vi "ggg.vi"() -> ()   [LabVIEW 2015]
uses:
  <vilib>/NXT/Block Support/NXT_InputPort.ctl
  <vilib>/NXT/Block Support/NXT_OutputPort.ctl
  <vilib>/NXT/Dual Mode Library/Sensors/Sonar_cm.vi
  <vilib>/NXT/Dual Mode Library/Sensors/Light_On.vi
  <vilib>/NXT/NXTIO Xnodes/NXTIONodeSubVIs/NXTMoveMotors.vi
  <vilib>/NXT/Dual Mode Library/Waits/Wait_Num.vi
  <vilib>/NXT/NXTIO Xnodes/AddressXNode/NXTIOAddress.xnode
  <vilib>/NXT/Subs/LVHSConnector.ctl
  <vilib>/NXT/NXTIO Xnodes/NXTIOXNode/NXTIO.xnode
  <vilib>/NXT/LegoClasses/BrickReference/BrickReference.lvclass
panel:
  in  "Port (Port 3) 4":T1=2 items=["Port 1", "Port 2", "Port 3", "Port 4"]
  in  "Port (Port 3) 3":T1=2 items=["Port 1", "Port 2", "Port 3", "Port 4"]
  in  "Power/Speed 1":i8=75
  in  "Port (Port 3) 2":T1=2 items=["Port 1", "Port 2", "Port 3", "Port 4"]
  in  "Port (Port 3)":T1=2 items=["Port 1", "Port 2", "Port 3", "Port 4"]
  in  "Power/Speed 3":i8=75
  in  "Port (Port 4)":T1=3 items=["Port 1", "Port 2", "Port 3", "Port 4"]
  in  "沥瘤":bool
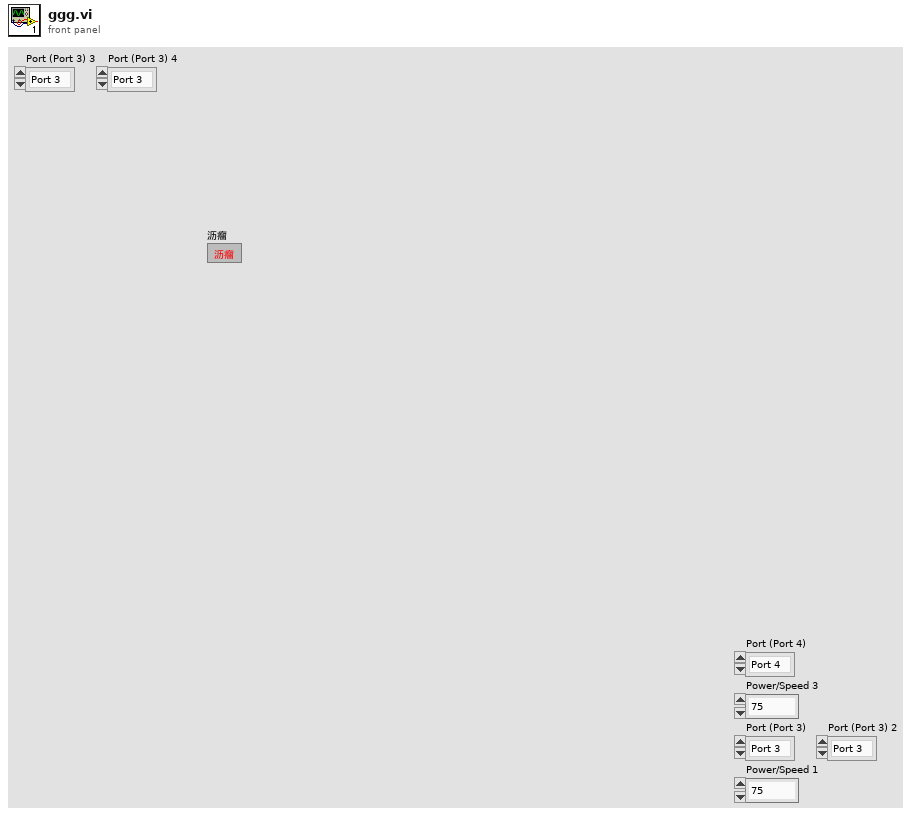
[diagram p1: front panel]
types:
  T1 = typedef "NXT_InputPort.ctl" = u32
  T2 = typedef "NXT_OutputPort.ctl" = u8
  T3 = cluster{"Output Port":T2, "Output Port 2":T2, "Output Port 3":T2}
  T4 = typedef "LVHSConnector.ctl" = refnum<class "BrickReference.lvclass">
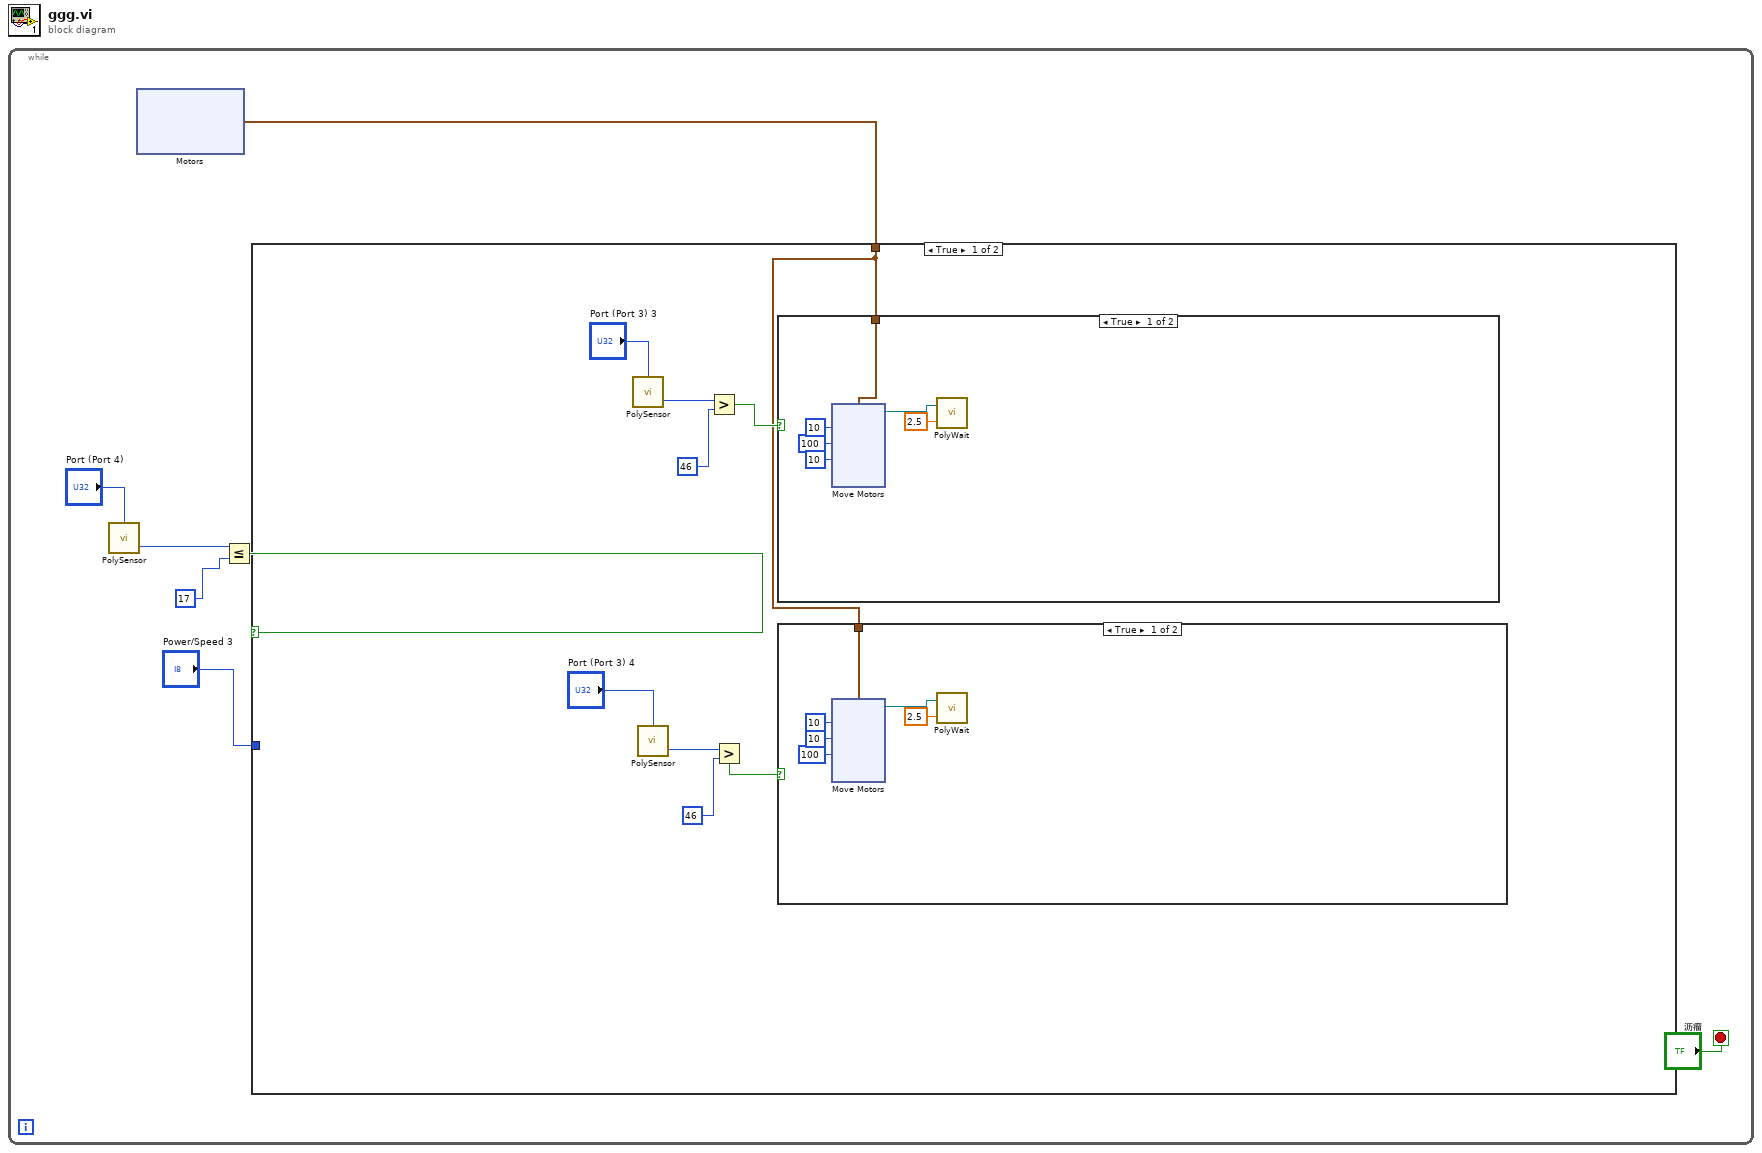
[diagram p0: block diagram]
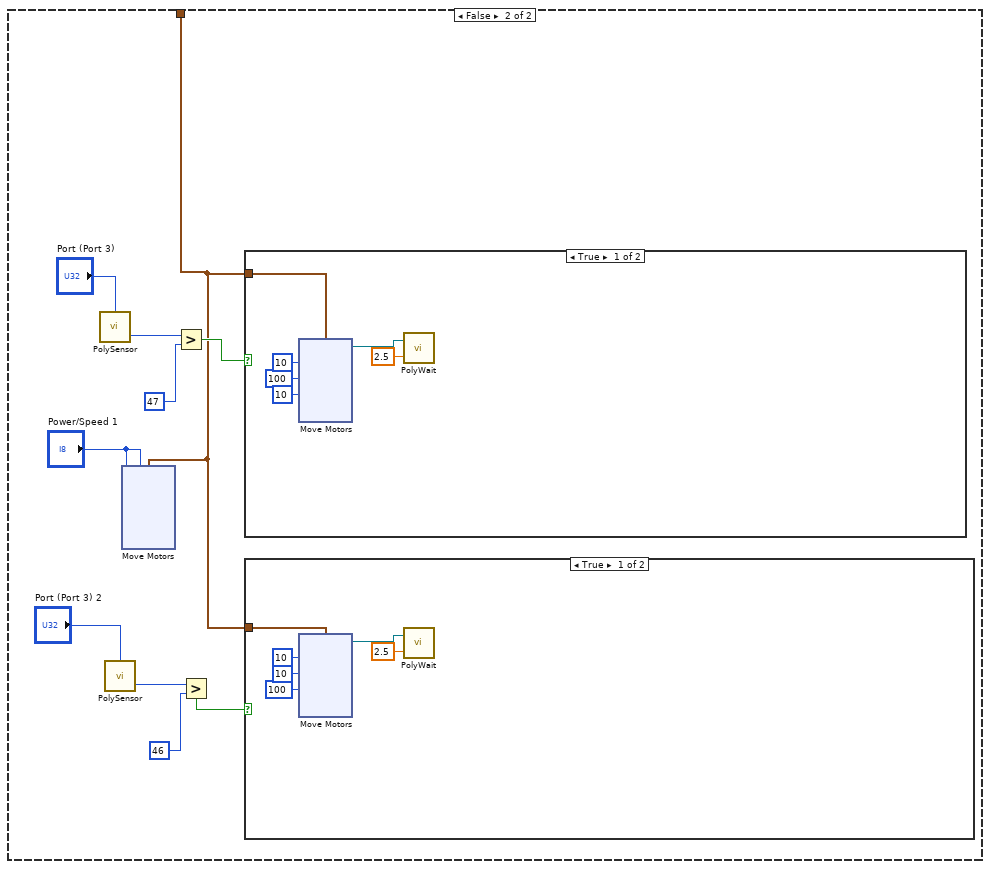
[diagram p4: hidden frame]
diagram:
  n1 = while {
    stop <- "沥瘤" stop-if-true
    n2 = call-poly <vilib>:"PolySensor.vi"("Port (Port 4)"="Port (Port 4)") -> ("Distance (cm)"=w4:i16)  [unwired: 2 in, 1 out]
    n3 = xnode "Motors"() -> ("Motor"=w1:cluster{"Port":T2, "Port":T2, "Port":T2})
    n4 = Less Or Equal?(x=w4, y=17) -> (x <= y?=w5:bool)
    n5 = case shown="True" w5 {
      tunnel: "Power/Speed 3" -> [_ _]
      tunnel: w1 -> [w9 w49]
      frame True {
        n6 = call-poly <vilib>:"PolySensor.vi"("Port (Port 3)"="Port (Port 3) 3") -> ("Scaled Value"=w14:i16)  [unwired: 2 in, 1 out]
        n7 = call-poly <vilib>:"PolySensor.vi"("Port (Port 3)"="Port (Port 3) 4") -> ("Scaled Value"=w17:i16)  [unwired: 2 in, 1 out]
        n8 = Greater?(x=w14, y=46) -> (0:w12:bool)
        n9 = Greater?(x=w17, y=46) -> (0:w15:bool)
        n10 = case shown="True" w12 {
          tunnel: w9 -> [w20 _]
          frame True {
            n11 = xnode "Move Motors"("Power/Speed 3"=i8 10, "Power/Speed 2"=i8 100, "Power/Speed 1"=i8 10, "Motors"=w20) -> ("NXT/EV3"=w23:T4)  [unwired: 1 in]
            n12 = call-poly <vilib>:"PolyWait.vi"("Time (1 sec)"=sgl 2.5, "NXT/EV3"=w23) -> ()  [unwired: 2 in, 1 out]
          }
          frame False {
          }
        }
        n13 = case shown="True" w15 {
          tunnel: w9 -> [w35 _]
          frame True {
            n14 = xnode "Move Motors"("Power/Speed 3"=i8 100, "Power/Speed 2"=i8 10, "Power/Speed 1"=i8 10, "Motors"=w35) -> ("NXT/EV3"=w38:T4)  [unwired: 1 in]
            n15 = call-poly <vilib>:"PolyWait.vi"("Time (1 sec)"=sgl 2.5, "NXT/EV3"=w38) -> ()  [unwired: 2 in, 1 out]
          }
          frame False {
          }
        }
      }
      frame False {
        n16 = call-poly <vilib>:"PolySensor.vi"("Port (Port 3)"="Port (Port 3)") -> ("Scaled Value"=w54:i16)  [unwired: 2 in, 1 out]
        n17 = call-poly <vilib>:"PolySensor.vi"("Port (Port 3)"="Port (Port 3) 2") -> ("Scaled Value"=w57:i16)  [unwired: 2 in, 1 out]
        n18 = xnode "Move Motors"("Power/Speed 3"="Power/Speed 1", "Power/Speed 2"="Power/Speed 1", "Power/Speed 1"="Power/Speed 1", "Motors"=w49) -> ()  [unwired: 1 in, 1 out]
        n19 = Greater?(x=w54, y=47) -> (0:w52:bool)
        n20 = Greater?(x=w57, y=46) -> (0:w55:bool)
        n21 = case shown="True" w52 {
          tunnel: w49 -> [w71 _]
          frame True {
            n22 = xnode "Move Motors"("Power/Speed 3"=i8 10, "Power/Speed 2"=i8 100, "Power/Speed 1"=i8 10, "Motors"=w71) -> ("NXT/EV3"=w72:T4)  [unwired: 1 in]
            n23 = call-poly <vilib>:"PolyWait.vi"("Time (1 sec)"=sgl 2.5, "NXT/EV3"=w72) -> ()  [unwired: 2 in, 1 out]
          }
          frame False {
          }
        }
        n24 = case shown="True" w55 {
          tunnel: w49 -> [w86 _]
          frame True {
            n25 = xnode "Move Motors"("Power/Speed 3"=i8 100, "Power/Speed 2"=i8 10, "Power/Speed 1"=i8 10, "Motors"=w86) -> ("NXT/EV3"=w87:T4)  [unwired: 1 in]
            n26 = call-poly <vilib>:"PolyWait.vi"("Time (1 sec)"=sgl 2.5, "NXT/EV3"=w87) -> ()  [unwired: 2 in, 1 out]
          }
          frame False {
          }
        }
      }
    }
  }
